vi "Status Update Core.vi"(8 "Error In":errorcluster, 10 "Log Message":T1={"Log Action"=enum."Handle Old Files", "Variant"=variant, "Data Type"=enum."String", "Group Name"="", "Channels Names"=[]}, 11 "TDMS Log In":refnum<class "TDMS Logger.lvclass">) -> (0 "Error Out":errorcluster)   [LabVIEW 2014, in "TDMS Logger.lvlib" / "TDMS Logger.lvclass"]
uses:
  TDMS Logger.lvclass
  _Typedefs/Log Message.ctl
  _Typedefs/Log Action.ctl
  _Typedefs/Data Type.ctl
  TDMS Logger.lvclass/TDMS Logger.ctl
  _Typedefs/Logger Status Information.ctl
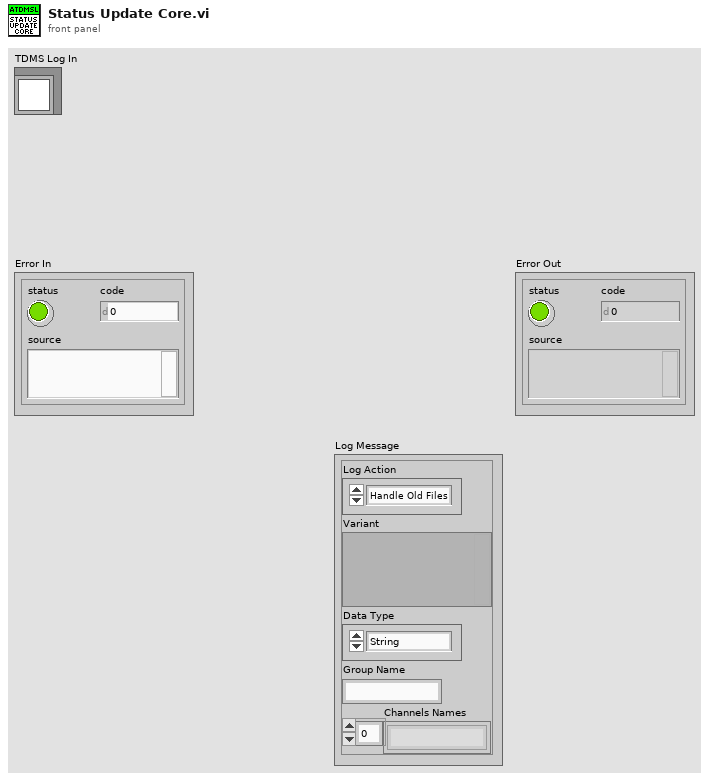
[diagram p1: front panel]
types:
  T1 = typedef "TDMS Logger.lvlib/TDMS Logger.lvclass/Log Message.ctl" = cluster{"Log Action":T2, "Variant":variant, "Data Type":T3, "Group Name":string, "Channels Names":string[]}
  T2 = typedef "TDMS Logger.lvlib/TDMS Logger.lvclass/Log Action.ctl" = enum16{"Handle Old Files", "Status Update", "Stop", "Log Data", "Initialize"}
  T3 = typedef "TDMS Logger.lvlib/TDMS Logger.lvclass/Data Type.ctl" = enum16{"I16", "I8", "String", "U16", "U8", "Waveform", "Double", "Single"}
  T4 = typedef "TDMS Logger.lvlib/TDMS Logger.lvclass/Logger Status Information.ctl" = cluster{"Number of Data Files":i32, "Current File Size (MB)":dbl, "Current Logs Path":path, "Last File Start":timestamp, "Throughput (MB/s)":dbl}
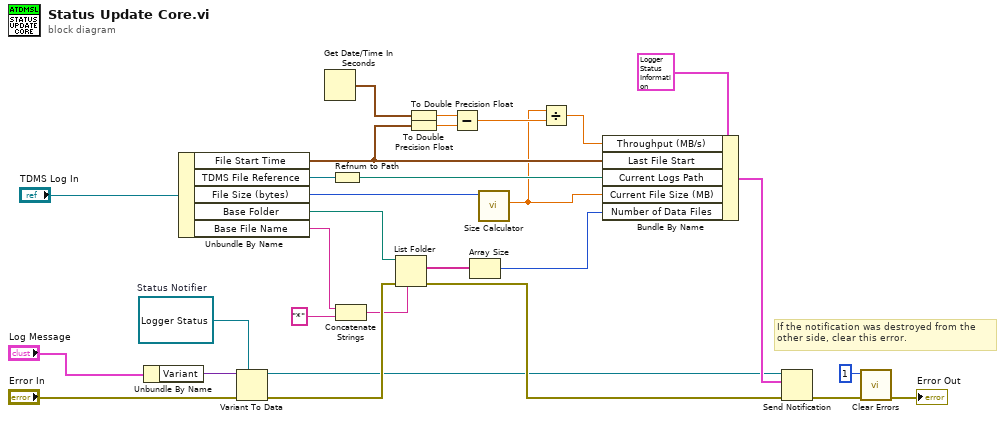
[diagram p0: block diagram]
diagram:
  w13 = refnum<notifier> refnum  # Status Notifier
  # "If the notification was destroyed from the\nother side, clear this error."
  n1 = Unbundle By Name("Log Message") -> ("Variant"=w12:variant)
  n2 = Unbundle By Name("TDMS Log In") -> ("File Start Time"=w9:timestamp, "TDMS File Reference"=w27:refnum<k34>, "File Size (bytes)"=w28:u64, "Base Folder"=w25:path, "Base File Name"=w18:string)
  n3 = Variant To Data(error in="Error In", type=w13, Variant=w12) -> (data=w14:refnum<notifier>, error out=w26:errorcluster)
  n4 = Get Date/Time In Seconds() -> (seconds since 1Jan1904=w10:timestamp)
  n5 = Refnum to Path(1:w27) -> (0:w17:path)
  n6 = Concatenate Strings(w18, "*" ("string")) -> (w22:string)
  n7 = List Folder(path=w25, pattern=w22, error in=w26) -> (filenames=w23:string[], error out=w29:errorcluster)  [unwired: 1 in, 2 out]
  n8 = To Double Precision Float(number=w10) -> (double precision float=w5:dbl)
  n9 = To Double Precision Float(number=w9) -> (double precision float=w4:dbl)
  n10 = Subtract(x=w5, y=w4) -> (x-y=w8:dbl)
  n11 = Array Size(array=w23) -> (size(s)=w24:i32)
  n12 = call "Size Calculator.vi"("Bytes"=w28) -> ("Megabytes"=w6:dbl)  [unwired: 8 in, 2 out]
  n13 = Divide(x=w6, y=w8) -> (x/y=w7:dbl)
  n14 = Bundle By Name(cluster=T4 {"Number of Data Files"=0, "Current File Size (MB)"=0.0, "Current Logs Path"=path "", "Last File Start"=timestamp(0 s since 1904-01-01), "Throughput (MB/s)"=0.0} ("notification"), "Throughput (MB/s)"=w7, "Last File Start"=w9, "Current Logs Path"=w17, "Current File Size (MB)"=w6, "Number of Data Files"=w24) -> (w20:T4)
  n15 = Send Notification(notification=w20, notifier=w14, error in (no error)=w29) -> (error out=w3:errorcluster)  [unwired: 1 out]
  n16 = call <vilib>:"Clear Errors.vi"("error in (no error)"=w3, "specific error code to clear (0: all)"=1) -> ("error out"=→"Error Out":errorcluster)  [unwired: 4 in, 1 out]
